vi "HMI.vi"(8 "error in (no error)":errorcluster caption="entrée d'erreur (pas d'erreur)", 11 "Class Popup Operator_Validation (Default) en entrée":refnum<class "Class Popup Result_Info.lvclass">) -> (0 "error out":errorcluster caption="sortie d'erreur", 1 "Input":string, 2 "Operator_Selection":bool, 3 "Class Popup Operator_Validation (Default) en sortie":refnum<class "Class Popup Result_Info.lvclass">)   [LabVIEW 2020, in "Library Instrument & Equipement.lvlib" / "Library Popup.lvlib" / "Class Popup Result_Info.lvclass"]
uses:
  Class Popup Result_Info.lvclass
  C:/Users/ngarcin/OneDrive - Altyor/Standard TB/Class/Popup/Class Popup (Main)/Class Popup (Main).lvclass
  C:/Users/ngarcin/OneDrive - Altyor/Standard TB/Class/Popup/Class Popup Result Information/Class Popup Result_Info (Virtual)/Class Popup Result_Info (Virtual).lvclass
  Class Popup Result_Info (Virtual)/Class Popup Result_Info (Virtual).lvclass
  Class Popup Result_Info.lvclass/Class Popup Result_Info.ctl
panel:
  in  "Bouton NOK":bool caption="Default"
  in  "Arbre Liste SN":string[](tree)
  in  "Bouton OK":bool caption="Validated"
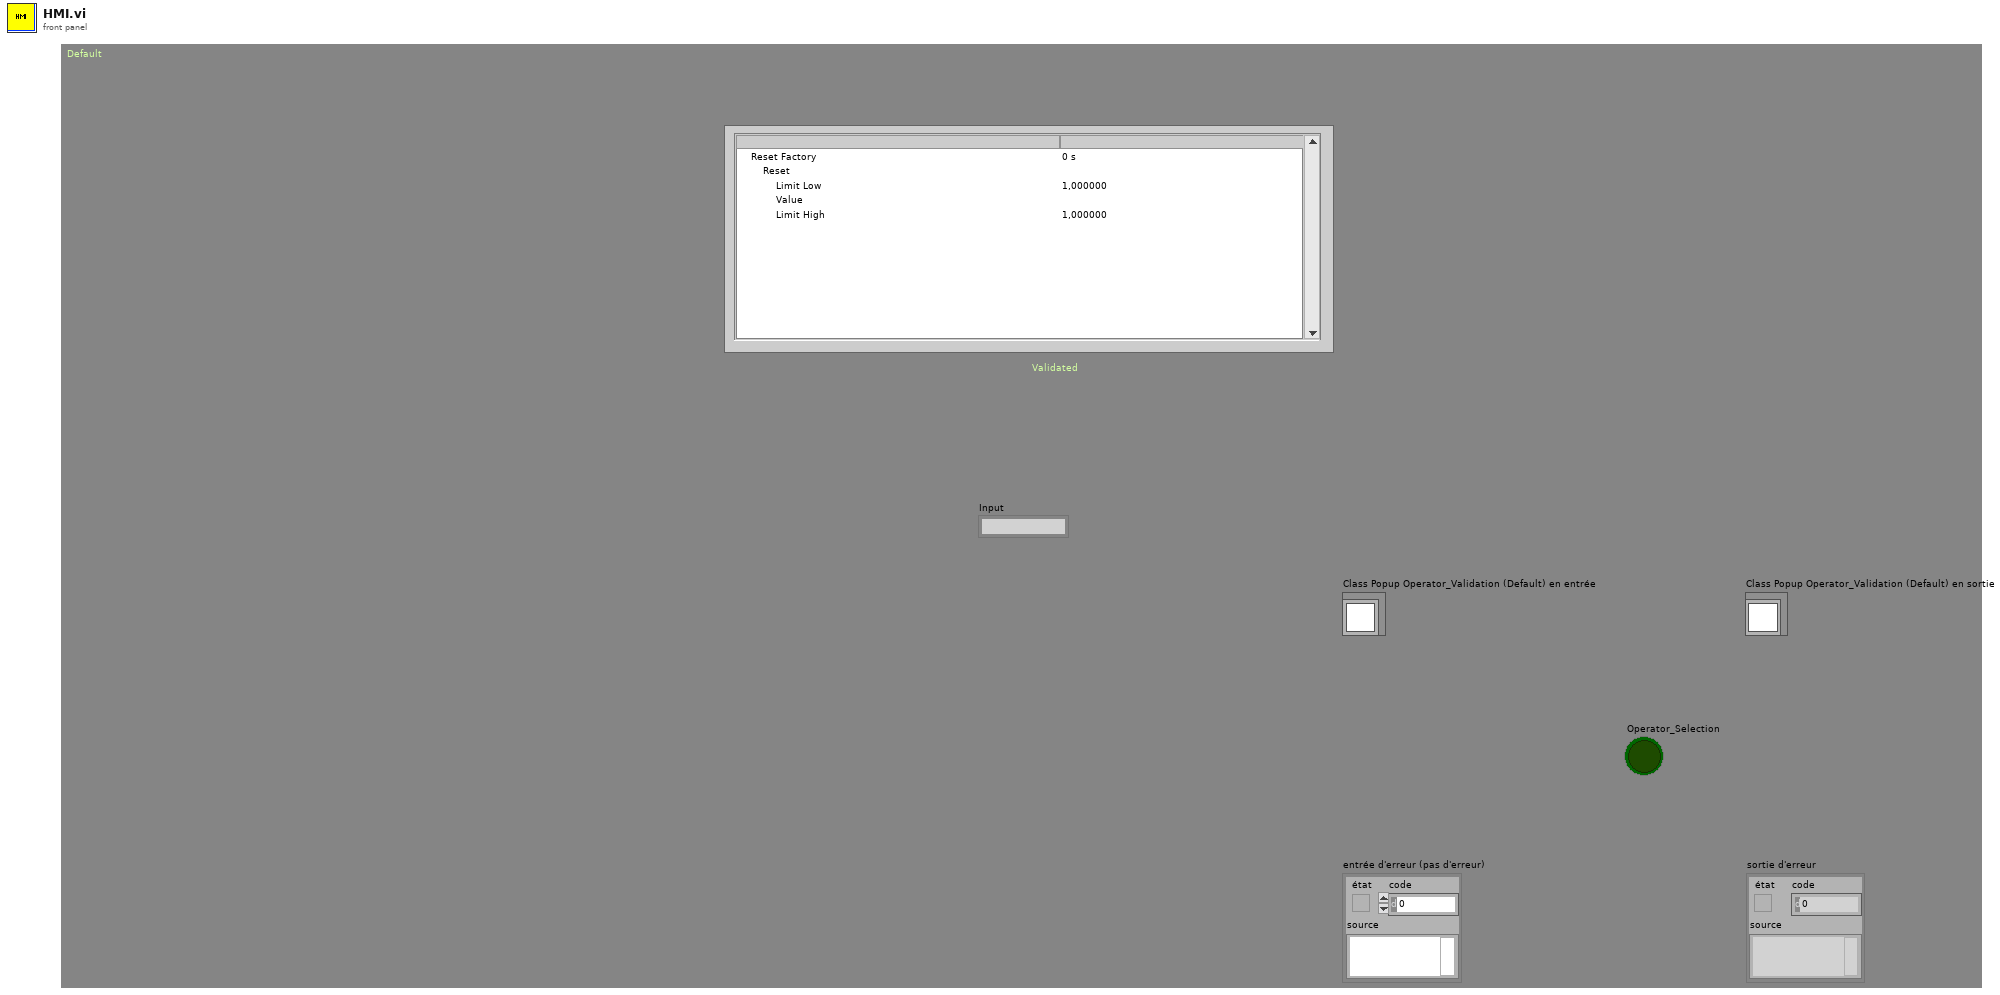
[diagram p1: front panel]
types:
  T1 = typedef "Library Commun.lvlib/Commande Value Type.ctl" = enum16{"None", "String", "Number", "Timestamp", "Boolean", "Array"}
  T2 = typedef "Library Commun.lvlib/Commande Type Test.ctl" = enum16{"Function", "Test", "Calculation"}
  T3 = cluster{"Main Test":string, "Name Test":string, "StartOfTest":string, "Value":string, "Limit_Low":string, "Limit_High":string, "Result":bool, "Fatal_Test":bool, "NbRetry":dbl, "EndOfTest":string, "Error":string, "TypeValue":T1, "Type Test":T2}[]
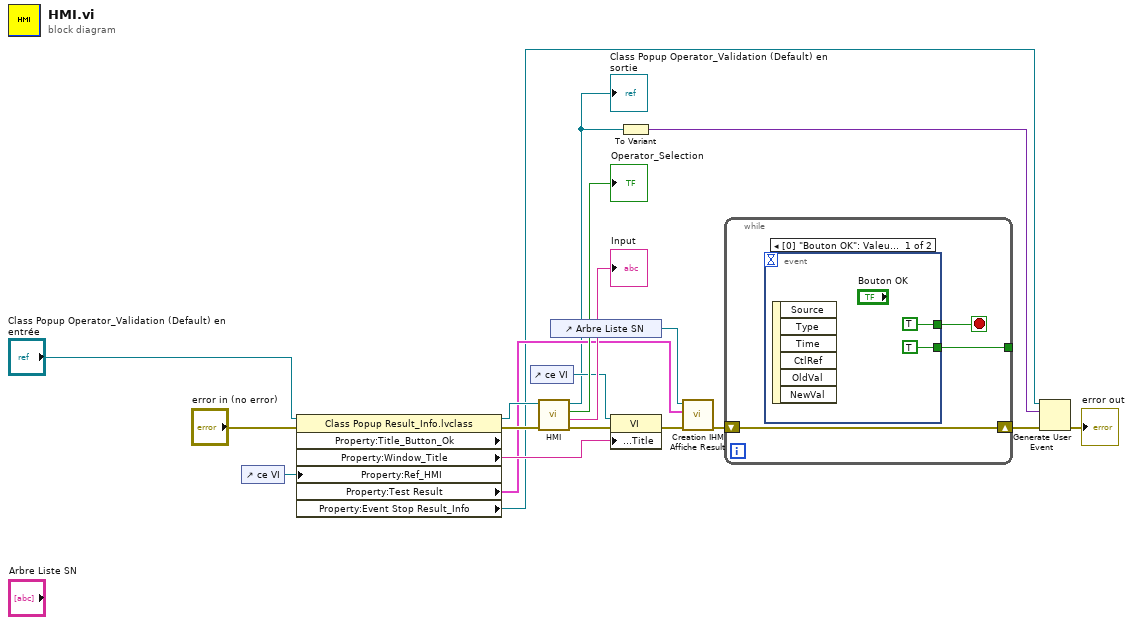
[diagram p0: block diagram]
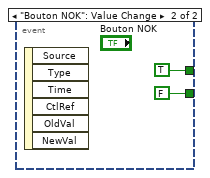
[diagram p2: hidden frame]
diagram:
  n1 = control-ref of="ce VI"() -> (w16:refnum<vi>)
  n2 = property class="Class Popup Result_Info.lvclass" props=["Property:Title_Button_Ok", "Property:Window_Title", "Property:Ref_HMI", "Property:Test Result", "Property:Event Stop Result_Info"](reference="Class Popup Operator_Validation (Default) en entrée", error in="error in (no error)", "Property:Ref_HMI"=w16) -> (reference out=w17:refnum<class "Class Popup Result_Info.lvclass">, error out=w18:errorcluster, "Property:Window_Title"=w19:string, "Property:Test Result"=w9:T3, "Property:Event Stop Result_Info"=w3:refnum<user-event>)  [unwired: 1 out]
  n3 = control-ref of="ce VI"() -> (w6:refnum<vi>)
  n4 = call-parent "HMI.vi"("error in (no error)"=w18, "Class Popup Operator_Validation (Default) en entrée"=w17) -> ("error out"=w11:errorcluster, "Input"=→"Input":string, "Operator_Selection"=→"Operator_Selection":bool, "Class Popup Operator_Validation (Default) en sortie"=w2:refnum<class "Class Popup Result_Info.lvclass">)  [unwired: 6 in]
  "Class Popup Operator_Validation (Default) en sortie" <- w2
  n5 = control-ref of="Arbre Liste SN"() -> (w5:refnum<vi>)
  n6 = property class="VI"(reference=w6, error in=w11, "Front Panel.Title"=w19) -> (error out=w8:errorcluster)  [unwired: 1 out]
  n7 = To Variant(anything=w2) -> (Variant=w1:variant)
  n8 = call "Creation IHM Affiche Result.vi"("error in (no error)"=w8, "Test Result"=w9, "Arbre Liste SN"=w5) -> ("error out"=w7:errorcluster)  [unwired: 8 in]
  n9 = while {
    tunnel: [w20] -> _
    shift-right: [w21] -> w10
    shift-left: w7 -> [w21]
    stop <- w22 stop-if-true
    n10 = event shown="[0] \"Bouton OK\": Valeur changée" {
      selector: _ -> [_ _]
      dyn-events: _ -> [_ _]
      timeout: _ -> [_ _]
      tunnel: [TRUE ("Valeur (Signalisation)") TRUE ("Valeur (Signalisation)")] -> w22
      tunnel: [TRUE ("Operator_Selection") FALSE ("Operator_Selection")] -> w20
      event "Bouton OK": Value Change {
        n11 = event-data() -> ()  [unwired: 1 in, 6 out]
      }
      event "Bouton NOK": Value Change {
        n12 = event-data() -> ()  [unwired: 1 in, 6 out]
      }
    }
  }
  n13 = Generate User Event(user event=w3, event data cluster=w1, error in=w10) -> (error out=→"error out":errorcluster)  [unwired: 1 in, 1 out]
